vi "Move Item.vi"(0 "Display State In":T1={"Prompt"="", "Listbox"=refnum, "Required"={"Strings"=[], "Bottom"=FALSE, "Italic"=FALSE, "FG"=0, "BG"=0, "Bold"=FALSE}, "Items"=[], "Req'd"=[], "Events"={"Items Changed"=refnum, "List Changed"=refnum}, "Max Rows"=-1, "Default name"=""}, 7 "Move from":i32, 11 "Move to":i32) -> (4 "Display State Out":T1={"Prompt"="", "Listbox"=refnum, "Required"={"Strings"=[], "Bottom"=FALSE, "Italic"=FALSE, "FG"=0, "BG"=0, "Bold"=FALSE}, "Items"=[], "Req'd"=[], "Events"={"Items Changed"=refnum, "List Changed"=refnum}, "Max Rows"=-1, "Default name"=""})   [LabVIEW 2015, in "KListboxEx.xctl"]
uses:
  KListboxEx.xctl
  State.ctl
  Required.ctl
  Events.ctl
  Event Action.ctl
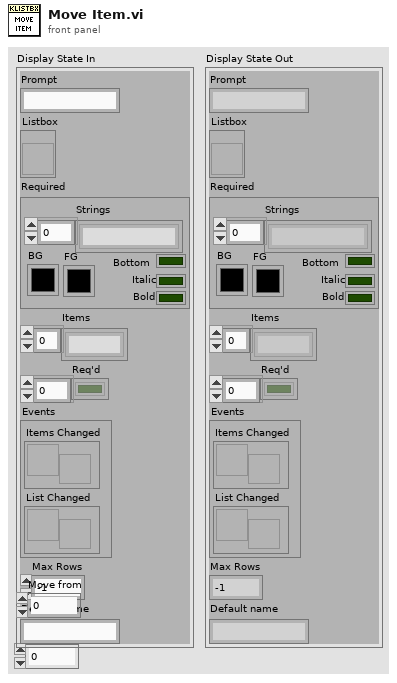
[diagram p1: front panel]
types:
  T1 = typedef "KListboxEx.xctl/State.ctl" = cluster{"Prompt":string, "Listbox":refnum<vi>, "Required":T2, "Items":string[], "Req'd":bool[], "Events":T3, "Max Rows":i32, "Default name":string}
  T2 = typedef "KListboxEx.xctl/Required.ctl" = cluster{"Strings":string[], "Bottom":bool, "Italic":bool, "FG":u32, "BG":u32, "Bold":bool}
  T3 = typedef "KListboxEx.xctl/Events.ctl" = cluster{"Items Changed":refnum<user-event>, "List Changed":refnum<user-event>}
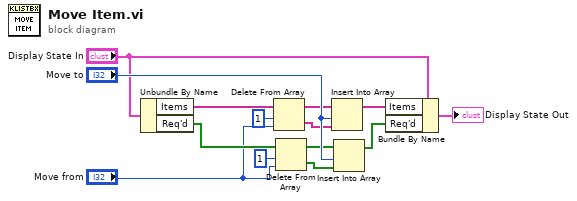
[diagram p0: block diagram]
diagram:
  n1 = Unbundle By Name("Display State In") -> ("Items"=w8:string[], "Req'd"=w9:bool[])
  n2 = Delete From Array(array=w8, length=1, index="Move from") -> (deleted portion=w2:string[], array with subset deleted=w3:string[])
  n3 = Delete From Array(array=w9, length=1, index="Move from") -> (deleted portion=w5:bool[], array with subset deleted=w6:bool[])
  n4 = Insert Into Array(array=w3, index="Move to", new element=w2) -> (w11:string[])
  n5 = Insert Into Array(array=w6, index="Move to", new element=w5) -> (w12:bool[])
  n6 = Bundle By Name(cluster="Display State In", "Items"=w11, "Req'd"=w12) -> (→"Display State Out":T1)
